vi "Get Power and Diagnostic Data.vi"() -> (2 "Power and Diagnostic Data":T1)   [LabVIEW 2014]
uses:
  Common Code/Power and Diagnostic Data.ctl
  Common Code/Utilities/PDP Data.ctl
  Common Code/Utilities/PCM Data.ctl
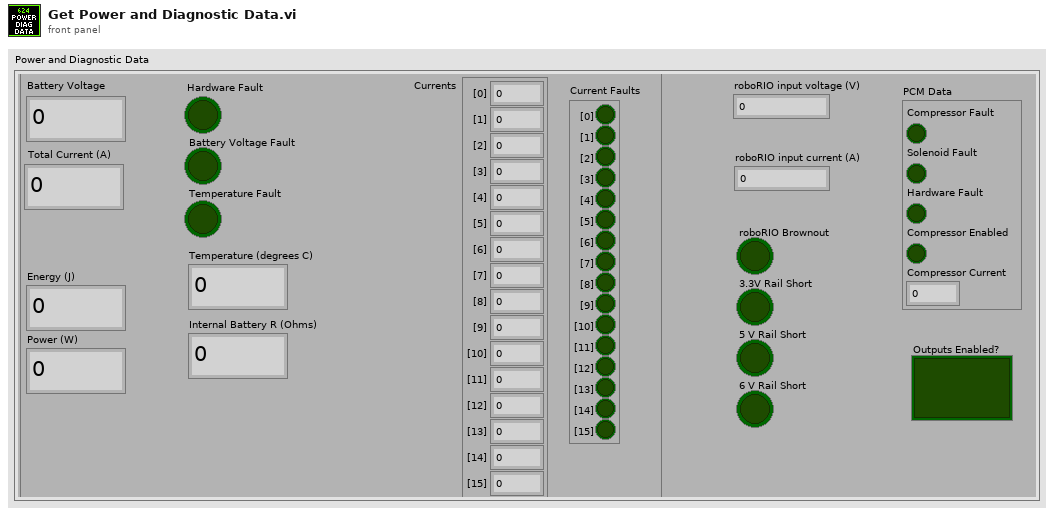
[diagram p1: front panel]
types:
  T1 = typedef "Power and Diagnostic Data.ctl" = cluster{"PDP Data":T2, "PCM Data":T3, "roboRIO input voltage (V)":dbl, "roboRIO input current (A)":dbl, "3.3V Rail Short":bool, "5 V Rail Short":bool, "6 V Rail Short":bool, "roboRIO Brownout":bool, "Outputs Enabled?":bool}
  T2 = typedef "PDP Data.ctl" = cluster{"Battery Voltage":dbl, "Temperature (degrees C)":dbl, "Internal Battery R (Ohms)":dbl, "Energy (J)":dbl, "Power (W)":dbl, "Total Current (A)":dbl, "Battery Voltage Fault":bool, "Temperature Fault":bool, "Hardware Fault":bool, "Currents":cluster{"[0]":dbl, "[1]":dbl, "[2]":dbl, "[3]":dbl, "[4]":dbl, "[5]":dbl, "[6]":dbl, "[7]":dbl, "[8]":dbl, "[9]":dbl, "[10]":dbl, "[11]":dbl, "[12]":dbl, "[13]":dbl, "[14]":dbl, "[15]":dbl}, "Current Faults":cluster{"[0]":bool, "[1]":bool, "[2]":bool, "[3]":bool, "[4]":bool, "[5]":bool, "[6]":bool, "[7]":bool, "[8]":bool, "[9]":bool, "[10]":bool, "[11]":bool, "[12]":bool, "[13]":bool, "[14]":bool, "[15]":bool}}
  T3 = typedef "PCM Data.ctl" = cluster{"Compressor Fault":bool, "Solenoid Fault":bool, "Compressor Enabled":bool, "Hardware Fault":bool, "Compressor Current":dbl}
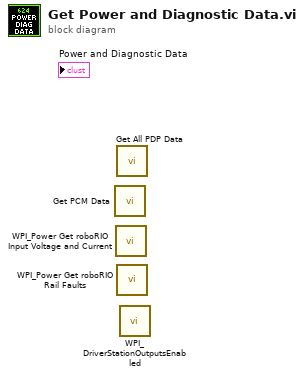
[diagram p0: block diagram]
diagram:
  n1 = call "Get PCM Data.vi"() -> ()  [unwired: 14 in, 2 out]
  n2 = call <vilib>:"WPI_Power Get roboRIO Input Voltage and Current.vi"() -> ()  [unwired: 13 in, 3 out]
  n3 = call "Get All PDP Data.vi"() -> ()  [unwired: 14 in, 2 out]
  n4 = call <vilib>:"WPI_Power Get roboRIO Rail Faults.vi"() -> ()  [unwired: 11 in, 5 out]
  n5 = call <vilib>:"WPI_DriverStationOutputsEnabled.vi"() -> ()  [unwired: 10 in, 2 out]
